vi "heating or cooling.vi"() -> ()   [LabVIEW 2015]
panel:
  in  "heating or cooling":u8
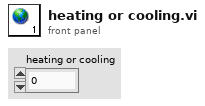
[diagram p1: front panel]
diagram:
